vi "Approximate Polygon.vi"   [LabVIEW 2020, in "shape.lvlib"]
doc: "Approximate a Polygon from a contour."
uses:
  shape.lvlib
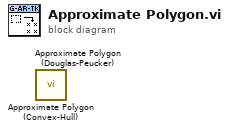
[diagram p0: block diagram]
diagram:
  n1 = call "Approximate Polygon (Convex-Hull).vi"() -> ()  [unwired: 10 in, 2 out]
  n2 = call "Approximate Polygon (Douglas-Peucker).vi"() -> ()  [unwired: 10 in, 2 out]
